vi "test.Create.TradeExpanded.vi"() -> (3 "Passed":bool)   [LabVIEW 2022 SP3]
uses:
  Trade/TradeExpanded.Parameters.ctl
  Trade/TradeExpanded.lvclass
panel:
  in  "TradeExpanded.Parameters":T1={"Time Offset"=447000, "Order Id"="ORID0001", "Quantity"=20000, "Symbol"="AAPL", "Side Indicator"="B", "Price"=0.905, "Execution Id"="EXE_ID_1"}
  out "x = y?":bool[](array[boolean])
  out "Python.Bytes.Out":u8[](array[numeric]) format="%.0x"
  out "LabVIEW.Bytes.Out":u8[](array[numeric]) format="%.0x"
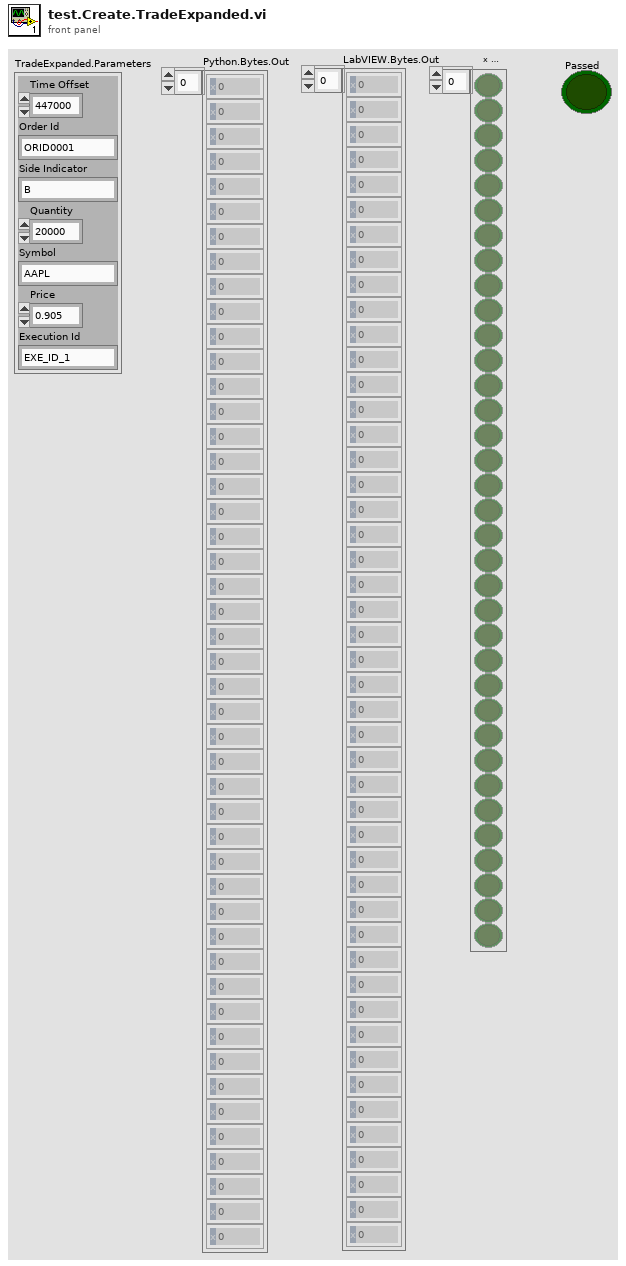
[diagram p1: front panel]
types:
  T1 = typedef "TradeExpanded.lvclass/TradeExpanded.Parameters.ctl" = cluster{"Time Offset":u32, "Order Id":string, "Quantity":u32, "Symbol":string, "Side Indicator":string, "Price":dbl, "Execution Id":string}
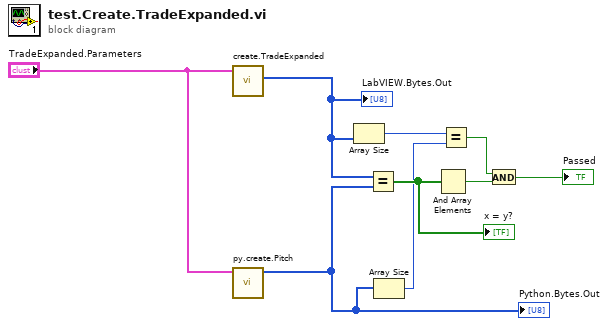
[diagram p0: block diagram]
diagram:
  n1 = call "create.TradeExpanded.vi"("TradeExpanded.Parmeters"="TradeExpanded.Parameters") -> ("Bytes.out"=w6:u8[])  [unwired: 9 in, 1 out]
  "LabVIEW.Bytes.Out" <- w6
  n2 = call "py.create.Pitch.vi"("Parameters"="TradeExpanded.Parameters") -> ("bytes"=w3:u8[])  [unwired: 9 in, 1 out]
  "Python.Bytes.Out" <- w3
  n3 = Array Size(array=w6) -> (size(s)=w4:i32)
  n4 = Equal?(x=w6, y=w3) -> (x = y?=w9:bool[])
  "x = y?" <- w9
  n5 = Array Size(array=w3) -> (size(s)=w2:i32)
  n6 = And Array Elements(Boolean array=w9) -> (logical AND=w7:bool)
  n7 = Equal?(x=w4, y=w2) -> (x = y?=w5:bool)
  n8 = And(x=w5, y=w7) -> (x .and. y?=→"Passed":bool)
